vi "TestDynamixelMultiturn.vi"() -> ()   [LabVIEW 2013]
uses:
  <instrlib>/Dynamixel Motor/Dynamixel Motor.lvlib
panel:
  out "Motors IDs Found":u8[](array[numeric])
  out "loop counter":i32
  in  "stop":bool
  in  "Goal Position (150 deg)":dbl=150.0
  in  "Motor ID (1)":u8=1
  in  "VISA resource name":refnum<visa-resource-name>="ASRL3::INSTR"
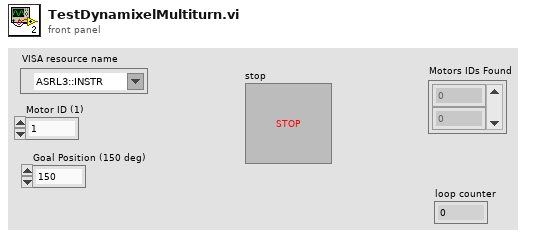
[diagram p1: front panel]
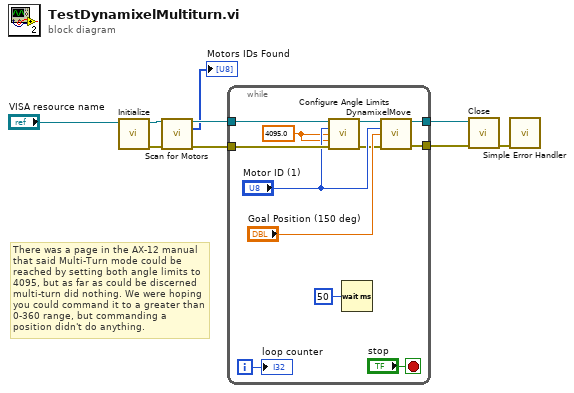
[diagram p0: block diagram]
diagram:
  # "There was a page in the AX-12 manual that said Multi-Turn mode could be reached by setting both angle limits to 4095, but as far as could be discerned multi-turn did nothing. We were hoping you could command it to a greater than 0-360 range, but commanding a position didn't do anything."
  n1 = call <instrlib>:"Initialize.vi"("VISA resource name"="VISA resource name") -> ("error out"=w8:errorcluster, "VISA resource name out"=w9:refnum<visa-resource-name>)  [unwired: 9 in]
  n2 = call <instrlib>:"Scan for Motors.vi"("VISA resource name"=w9, "error in (no error)"=w8) -> ("VISA resource name out"=w6:refnum<visa-resource-name>, "Motors IDs Found"=→"Motors IDs Found":u8[], "error out"=w5:errorcluster)  [unwired: 11 in]
  n3 = while {
    tunnel: w6 -> [w21]
    tunnel: w5 -> [w20]
    tunnel: [w16] -> w4
    tunnel: [w15] -> w2
    i -> [w12]
    stop <- "stop" stop-if-true
    w10 = 4095.0 ("Counter-Clockwise Angle Limit (300 deg)")
    n4 = call <instrlib>:"Configure Angle Limits.vi"("VISA resource name"=w21, "Motor ID (0)"="Motor ID (1)", "Clockwise Angle Limit (0 deg)"=w10, "Counter-Clockwise Angle Limit (300 deg)"=w10, "error in (no error)"=w20) -> ("VISA resource name out"=w19:refnum<visa-resource-name>, "error out"=w14:errorcluster)  [unwired: 9 in]
    n5 = Wait (ms)(milliseconds to wait=u32 50) -> ()  [unwired: 1 out]
    n6 = call "DynamixelMove.vi"("VISA resource name"=w19, "Motor ID (0)"="Motor ID (1)", "Goal Position (150 deg)"="Goal Position (150 deg)", "error in (no error)"=w14) -> ("VISA resource name out"=w16:refnum<visa-resource-name>, "error out"=w15:errorcluster)  [unwired: 10 in]
    "loop counter" <- w12
  }
  n7 = call <instrlib>:"Close.vi"("error in (no error)"=w2, "VISA resource name"=w4) -> ("error out"=w1:errorcluster)  [unwired: 9 in]
  n8 = call <vilib>:"Simple Error Handler.vi"("error in (no error)"=w1) -> ()  [unwired: 4 in, 5 out]
